vi "Flatten.vi"(8 "error in (no error)":errorcluster, 11 "anritsu reader in":refnum<class "anritsu reader.lvclass">) -> (0 "error out":errorcluster, 3 "anritsu reader out":refnum<class "anritsu reader.lvclass">)   [LabVIEW 2023, in "anritsu reader.lvclass"]
uses:
  anritsu reader.lvclass
  anritsu reader.lvclass/anritsu reader.ctl
  Global/File Locations.vi
  Reader/Reader.lvclass
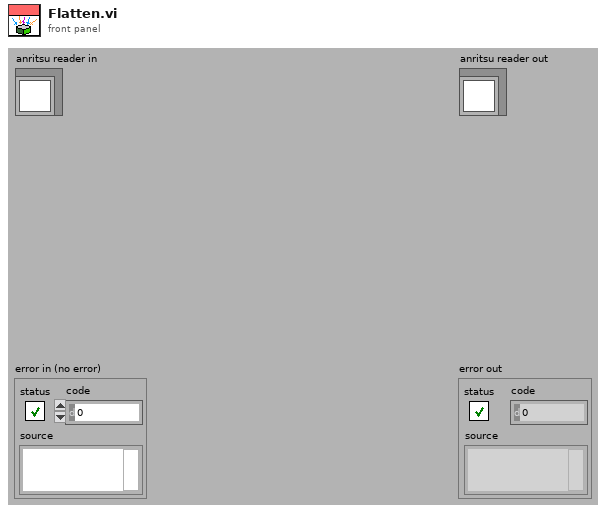
[diagram p1: front panel]
types:
  T1 = typedef "Anritsu Power Meter.lvlib/Averaging control.ctl" = enum16{"On", "Off"}
  T2 = typedef "Anritsu Power Meter.lvlib/Display control.ctl" = enum16{"Watt", "dBm", "dB (REL)"}
  T3 = typedef "Anritsu Power Meter.lvlib/Measuring rate control.ctl" = enum16{"Hold", "Free Run", "Exit Trigger"}
  T4 = typedef "Anritsu Power Meter.lvlib/Range control watts and dBm.ctl" = enum16{"10 mW (+10 dBm)", "1 mW (0 dBm)", "100 uW (-10 dBm)", "10 uW (-20 dBm)", "1 uW (-30 dBm)", "100 nW (-40 dBm)", "10 nW (-50 dBm)", "1 nW (-60 dBm)", "100 pW (-70 dBm)", "10 pW (-80 dBm)"}
  T5 = typedef "Anritsu Power Meter.lvlib/Auto Range control.ctl" = enum16{"Off", "On"}
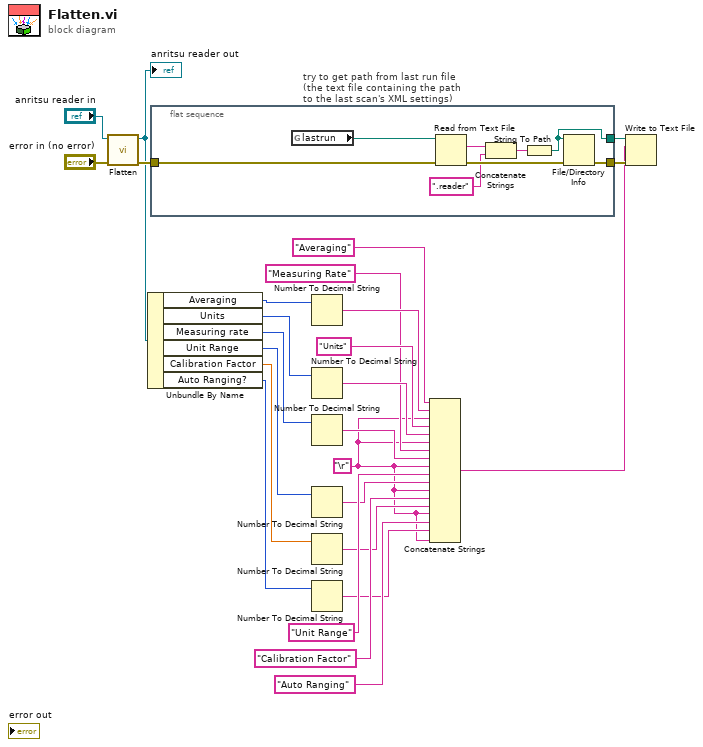
[diagram p0: block diagram]
diagram:
  w2 = "\r"
  n1 = call-parent "Flatten.vi"("error in (no error)"="error in (no error)", "Reader in"="anritsu reader in") -> ("error out"=w24:errorcluster, "Reader out"=w21:refnum<class "anritsu reader.lvclass">)  [unwired: 8 in]
  "anritsu reader out" <- w21
  n2 = Unbundle By Name(w21) -> ("Averaging"=w20:T1, "Units"=w19:T2, "Measuring rate"=w18:T3, "Unit Range"=w17:T4, "Calibration Factor"=w16:dbl, "Auto Ranging?"=w15:T5)
  n3 = flat-sequence "try to get path from last run file\n(the text file containing the path\nto the last scan's XML settings)" {
    tunnel: [w34] -> w22
    tunnel: [w31] -> w23
    tunnel: w24 -> [w30]
    frame #0 {
      n4 = global read "File Locations.vi" "lastrun"() -> (w33:path)
      n5 = Read from Text File(file (use dialog)=w33, error in=w30) -> (text=w29:string, error out=w32:errorcluster)  [unwired: 4 out]
      n6 = Concatenate Strings(w29, ".reader") -> (w27:string)
      n7 = String To Path(string=w27) -> (path=w34:path)
      n8 = File/Directory Info(path=w34, error in=w32) -> (error out=w31:errorcluster)  [unwired: 6 out]
    }
  }
  n9 = Number To Decimal String(number=w20) -> (decimal integer string=w13:string)  [unwired: 1 in]
  n10 = Number To Decimal String(number=w19) -> (decimal integer string=w11:string)  [unwired: 1 in]
  n11 = Number To Decimal String(number=w18) -> (decimal integer string=w6:string)  [unwired: 1 in]
  n12 = Number To Decimal String(number=w17) -> (decimal integer string=w5:string)  [unwired: 1 in]
  n13 = Number To Decimal String(number=w16) -> (decimal integer string=w4:string)  [unwired: 1 in]
  n14 = Number To Decimal String(number=w15) -> (decimal integer string=w3:string)  [unwired: 1 in]
  n15 = Concatenate Strings("Averaging", w13, w2, "Units", w11, w2, "Measuring Rate", w6, w2, "Unit Range", w5, w2, "Calibration Factor", w4, w2, "Auto Ranging", w3, w2) -> (w1:string)
  n16 = Write to Text File(file (use dialog)=w22, text=w1, error in=w23) -> ()  [unwired: 1 in, 3 out]
